vi "Subvi AO scan galvo.vi"(2 "AOmon":refnum<k21>="Connector1/AO1", 3 "AO":refnum<k21>="Connector1/AO0", 9 "FIFO":refnum<k21>="GALVO1") -> (0 "AOstateMon":u16)   [LabVIEW 2017]
uses:
  <vilib>/Platform/TimedLoop/XDataNode/timing_clust.ctl
  <vilib>/Platform/TimedLoop/XDataNode/nitl_modes.ctl
  <vilib>/Platform/TimedLoop/XDataNode/wakeup.ctl
  <vilib>/rvi/Emulation/niFpgaSctlEmulationGetInTimedLoop.vi
  <vilib>/rvi/Emulation/niFpgaEmulationReportErrorSimple.vi
  <vilib>/rvi/Emulation/niFpgaGetClockAttributes.vi
  <vilib>/rvi/Emulation/niFpgaCriticalErrorInLSC.vi
  GV scan galvo delay.vi
  GV preframegate.vi
  <vilib>/rvi/DataTransferAndStorage/Container/Common/niFpgaContainerExecOnDevCompGetState.vi
  <vilib>/rvi/Emulation/niFpgaEmulationIsFPGAContextNoSignature.vi
  <vilib>/rvi/DataTransferAndStorage/Container/Common/niFpgaContainerGetUniqueNameForEmu.vi
  <vilib>/rvi/Emulation/niFpgaProcessEmulError.vi
  <vilib>/rvi/errors/nirviReportUnexpectedCaseInternalError (U32).vi
  <vilib>/rvi/Memory/Memory_Emulation/niFpgaMemoryEmulationCacheClearOnFirstRun.vi
  <vilib>/rvi/Memory/Memory_Emulation/nirvimemoryEmulationManagerCache_MakeExclusive.vi
  <vilib>/rvi/Memory/Memory_Emulation/niFpgaMemoryEmulationValidateCache.vi
  <vilib>/rvi/Memory/Memory_Emulation/nirvimemoryEmulationManagerCache_InsertValue.vi
  <vilib>/Utility/error.llb/Clear Errors.vi
  <vilib>/rvi/Memory/Memory_Emulation/nirvimemoryEmulationManagerCache_ReleaseExclusive.vi
  <vilib>/rvi/Memory/Memory_Emulation/nirvimemoryEmulationManagerCache_GetValue.vi
  <vilib>/rvi/Memory/Memory_Emulation/nirvimemoryEmulationManagerCache_SetValue.vi
  <vilib>/rvi/Emulation/niFpgaSctlEmulationResourceMgr.vi
  <vilib>/rvi/eio/common/nirviEmuTemplateMethod_errors.vi
  <vilib>/Platform/TimedLoop/XDataNode/XDataNode.xnode
  <vilib>/rvi/DataTransferAndStorage/Container/XNode/niFpgaContainer.xnode
  <vilib>/rvi/Memory/Memory_Emulation/niFpgaMemoryEmulationRefIn.vi
  <vilib>/eio/EIONode/EIONode.xnode
  <vilib>/Platform/TimedLoop/XDataNode/XDNodeRunTimeDep.lvlib
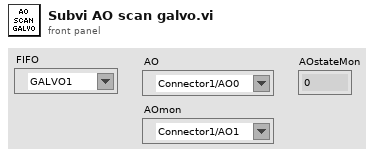
[diagram p1: front panel]
types:
  T1 = typedef "XDNodeRunTimeDep.lvlib/timing_clust.ctl" = cluster{"Expected End [f-1]":u64, "Actual End [f-1]":u64, "Finished Late? [f-1]":bool, "Expected End [i-1]":u64, "Actual End [i-1]":u64, "Finished Late? [i-1]":bool, "Expected Start [i]":u64, "Actual Start [i]":u64, "Expected Start [f]":u64, "Actual Start [f]":u64, "Source Name":string, "Structure Name":string, "Period":i64, "Deadline":i64, "Offset":i64, "Start":i64, "Priority":i32, "Timeout":i32, "Mode":T2, "Wakeup Reason":T3, "Error":errorcluster, "Source Type":string, "Secondary Source Type":string, "Global End Time":u64, "Global Start Time":u64, "Frame Duration":u64, "Iteration Duration":u64, "Assigned CPU":i32, "I/O Scan Engine Mode":u32}
  T2 = typedef "XDNodeRunTimeDep.lvlib/nitl_modes.ctl" = enum32{"No Change", "Process missed periods, maintain original phase", "Discard missed periods, maintain original phase", "Process missed periods, ignore original phase", "Discard missed periods, ignore original phase"}
  T3 = typedef "XDNodeRunTimeDep.lvlib/wakeup.ctl" = enum32{"Normal", "Aborted", "Asynchronous wakeup", "Timing source error", "Timed loop error", "Timeout"}
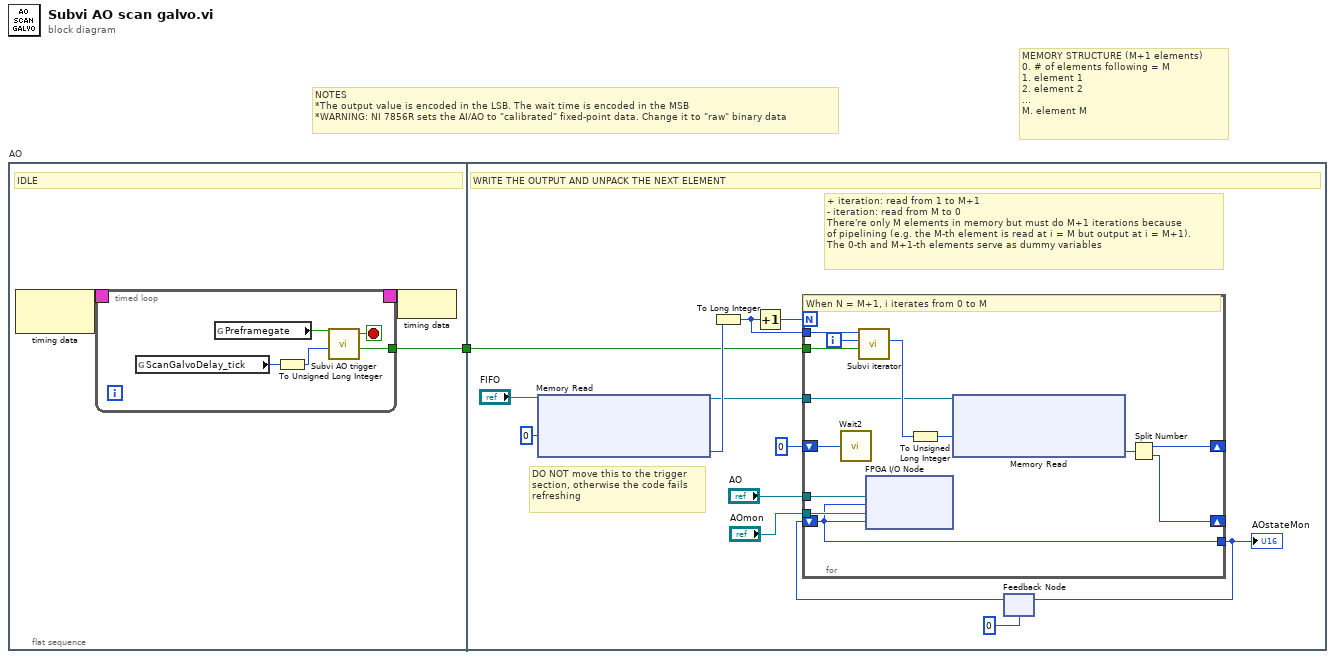
[diagram p0: block diagram]
diagram:
  # "MEMORY STRUCTURE (M+1 elements)\n0. # of elements following = M\n1. element 1\n2. element 2\n...\nM. element M"
  # "NOTES\n*The output value is encoded in the LSB. The wait time is encoded in the MSB\n*WARNING: NI 7856R sets the AI/AO to \"calibrated\" fixed-point data. Change it to \"raw\" binary data"
  n1 = flat-sequence "AO" {
    tunnel: [w4] -> w1
    tunnel: w1 -> [w19]
    frame #0 {
      # "IDLE"
      n2 = node-c288() -> (w3:T1)  [unwired: 1 in]
      n3 = timed-loop {
        timing: w3 -> [_]
        timing-out: [_] -> w2
        tunnel: [w8] -> w4
        stop <- w9 stop-if-true
        n4 = global read "GV scan galvo delay.vi" "ScanGalvoDelay_tick"() -> (w7:u16)
        n5 = global read "GV preframegate.vi" "Preframegate"() -> (w5:bool)
        n6 = To Unsigned Long Integer(number=w7) -> (unsigned 32bit integer=w6:u32)
        n7 = call "Subvi AO trigger.vi"("Delay_ticks"=w6, "Trigger"=w5) -> ("IteratorDirection"=w8:bool, "Stop"=w9:bool)  [unwired: 8 in]
      }
      n8 = node-c288(w2) -> ()
    }
    frame #1 {
      # "+ iteration: read from 1 to M+1\n- iteration: read from M to 0\nThere're only M elements in memory but must do M+1 iterations because \nof pipelining (e.g. the M-th element is read at i = M but output at i = M+1).\nThe 0-th and M+1-th elements serve as dummy variables"
      # "DO NOT move this to the trigger\nsection, otherwise the code fails\nrefreshing"
      # "WRITE THE OUTPUT AND UNPACK THE NEXT ELEMENT"
      n9 = xnode ("Memory Read")("Address"=u32 0, "Memory In"="FIFO") -> ("Data"=w25:u32, "Memory Out"=w24:refnum<k21>)
      n10 = To Long Integer(number=w25) -> (32bit integer=w17:i32)
      n11 = Increment(x=w17) -> (x+1=w18:i32)
      n12 = feedback #1(u16 0) -> (w15:u16)
      n13 = for {
        N: w18 -> [_]
        shift-right: [w37] -> _
        shift-left: u16 0 -> [w35]
        shift-right: [w36] -> _
        shift-left: w15 -> [w27]
        tunnel: [w27] -> w16
        tunnel: w17 -> [w32]
        tunnel: w24 -> [w31]
        tunnel: "AO" -> [w28]
        tunnel: w19 -> [w30]
        tunnel: "AOmon" -> [w29]
        i -> [w33]
        # "When N = M+1, i iterates from 0 to M"
        n14 = call "Wait2"("Count(Ticks)"=w35) -> ()  [unwired: 1 out]
        n15 = call "Subvi iterator.vi"("Set increase"=w30, "Iterator in"=w33, "Nmax"=w32) -> ("Iterator out"=w34:i32)  [unwired: 8 in]
        n16 = xnode ("FPGA I/O Node")("I/O Item"=w27, "FPGA I/O In"=w28, "I/O Item"=w27, "FPGA I/O In"=w29) -> ()  [unwired: 2 out]
        n17 = To Unsigned Long Integer(number=w34) -> (unsigned 32bit integer=w39:u32)
        n18 = xnode ("Memory Read")("Address"=w39, "Memory In"=w31) -> ("Data"=w38:u32)  [unwired: 1 out]
        n19 = Split Number(x=w38) -> (hi(x)=w37:u16, lo(x)=w36:u16)
      }
      "AOstateMon" <- w16
      n20 = feedback-in #1(w16) -> ()
    }
  }
